vi "libssh2_sftp_fsetstat.vi"(8 "error in (no error)":errorcluster, 10 "attributes":T1, 11 "sftp handle":T2) -> (0 "error out":errorcluster)   [LabVIEW 2013, in "libssh2.lvlib"]
doc: "Set file status."
uses:
  libssh2.lvlib
  SFTP Handle Refnum.ctl
  libssh2_sftp_attributes.ctl
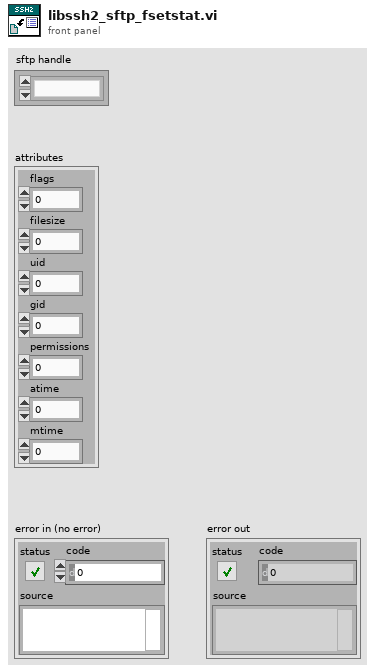
[diagram p1: front panel]
types:
  T1 = typedef "libssh2.lvlib/libssh2_sftp_attributes.ctl" = cluster{"flags":u32, "filesize":u64, "uid":u32, "gid":u32, "permissions":u32, "atime":u32, "mtime":u32}
  T2 = typedef "libssh2.lvlib/SFTP Handle Refnum.ctl" = refnum<k1>
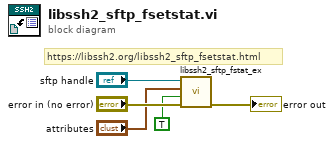
[diagram p0: block diagram]
diagram:
  # "https://libssh2.org/libssh2_sftp_fsetstat.html"
  n1 = call "libssh2_sftp_fstat_ex.vi"("error in (no error)"="error in (no error)", "set"=TRUE, "attributes"="attributes", "sftp handle"="sftp handle") -> ("error out"=→"error out":errorcluster)  [unwired: 6 in, 1 out]
